vi "Start Sync.vi"(8 "error in (no error)":errorcluster, 11 "gRPC Server in":refnum<class "Query Server.lvclass">) -> (0 "error out":errorcluster, 3 "gRPC Server out":refnum<class "Query Server.lvclass">)   [LabVIEW 2019, in "Query Server.lvlib" / "Query Server.lvclass"]
uses:
  Query Server.lvclass
  gRPC lvSupport/Server API/typeDefs/grpcId.ctl
  Query Server.lvclass/Query Server.ctl
  RPC Messages/ServerEvent/ServerEvent_Data.ctl
  gRPC lvSupport/gprc-lvsupport.lvlib
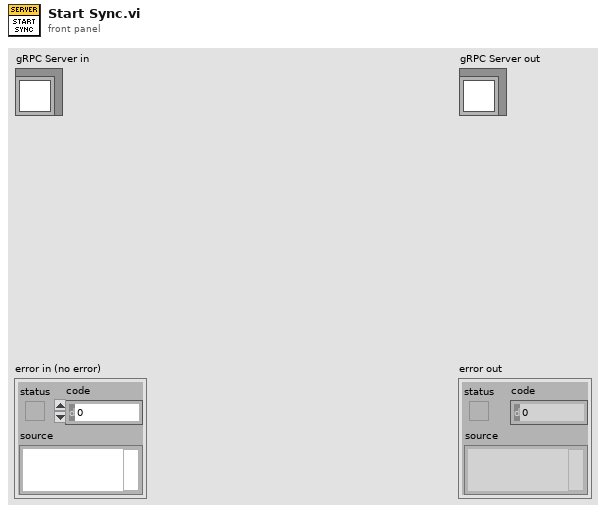
[diagram p1: front panel]
types:
  T1 = typedef "Query Server.lvlib/gprc-lvsupport.lvlib/grpcId.ctl" = u64
  T2 = typedef "Query Server.lvlib/Query Server.lvclass/ServerEvent_Data.ctl" = cluster{"eventData":string, "serverId":i32, "status":i32}
  T3 = typedef "Query Server.lvlib/Query Server.lvclass/Server gRPC UEs.ctl" = cluster{"Generic Method Event":refnum<user-event>}
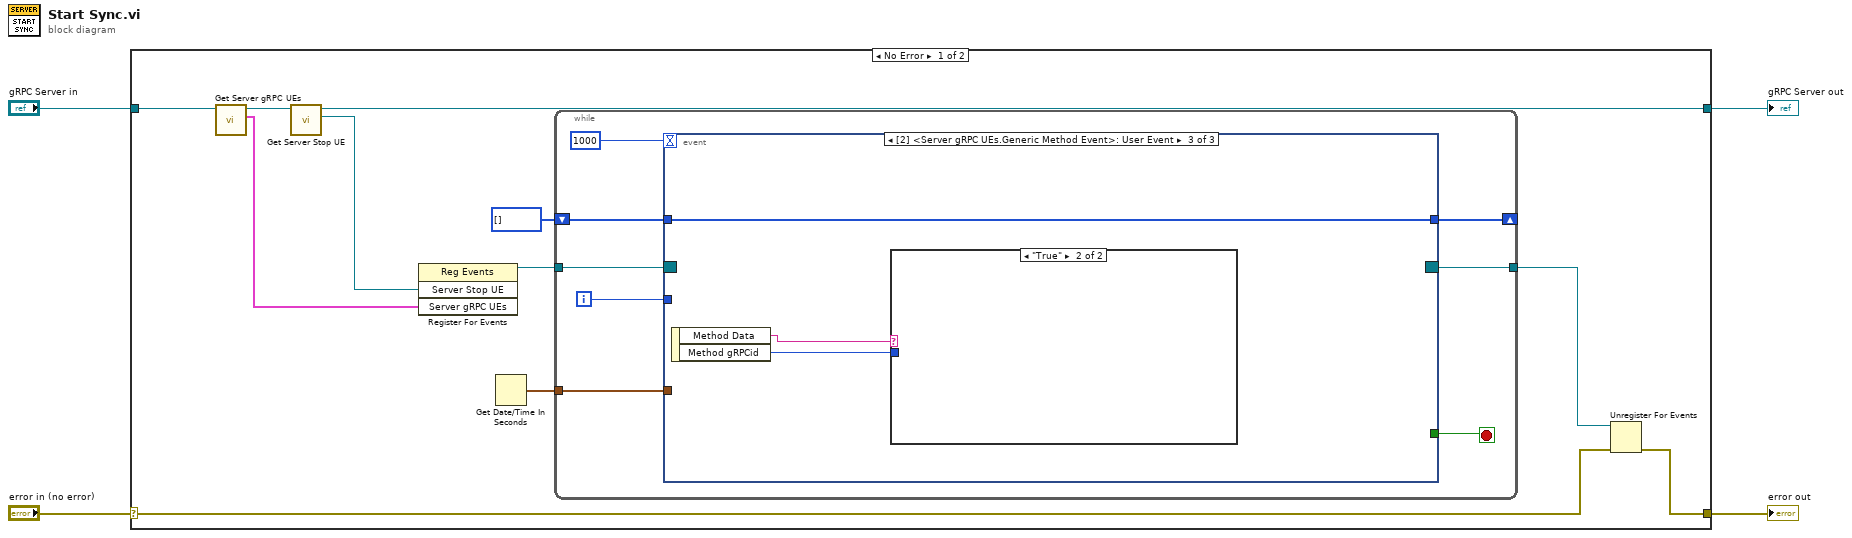
[diagram p0: block diagram]
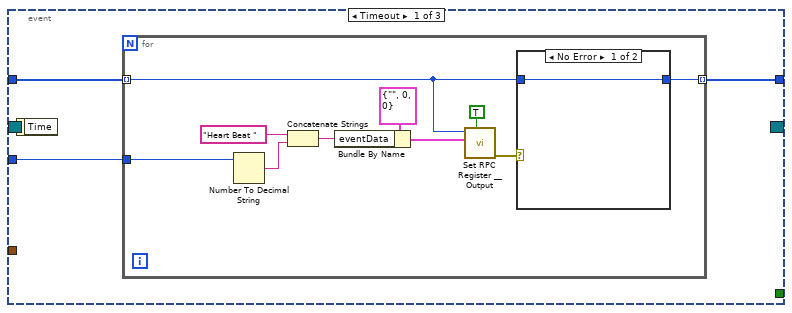
[diagram p2: hidden frame]
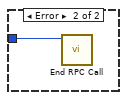
[diagram p3: hidden frame]
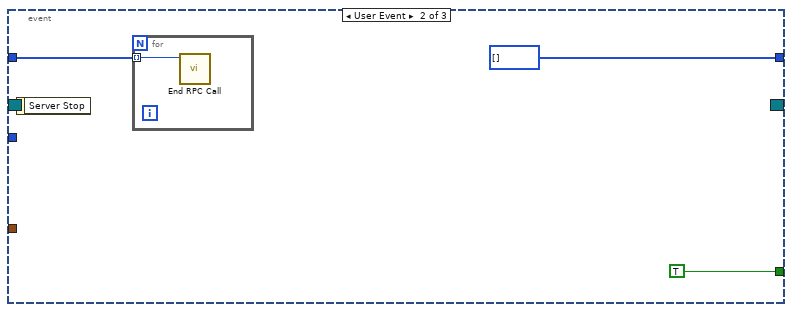
[diagram p4: hidden frame]
diagram:
  n1 = case shown="No Error" "error in (no error)" {
    selector: "error in (no error)" -> [w8 w47]
    tunnel: [w7 w47] -> w3
    tunnel: [w11 w46] -> w1
    tunnel: "gRPC Server in" -> [w15 w46]
    frame No Error {
      n2 = call "Get Server gRPC UEs.vi"("OOP Server in"=w15) -> ("Server gRPC UEs"=w12:T3, "OOP Server out"=w14:refnum<class "Query Server.lvclass">)  [unwired: 9 in]
      n3 = call "Get Server Stop UE.vi"("OOP Server in"=w14) -> ("Server Stop UE"=w13:refnum<user-event>, "OOP Server out"=w11:refnum<class "Query Server.lvclass">)  [unwired: 9 in]
      n4 = register-events(w13, w12) -> (reference out=w10:refnum<event-registration>)  [unwired: 2 in, 1 out]
      n5 = Get Date/Time In Seconds() -> (seconds since 1Jan1904=w6:timestamp)
      n6 = while {
        tunnel: w10 -> [w23]
        tunnel: [w21] -> w9
        shift-right: [w19] -> _
        shift-left: T1[] [] -> [w18]
        tunnel: w6 -> [w16]
        i -> [w17]
        stop <- w22 stop-if-true
        n7 = event "RPC Methods Event Structure" shown="[2] <Server gRPC UEs.Generic Method Event>: User Event" {
          selector: w23 -> [_ _ _]
          dyn-events: [_ _ _] -> w21
          timeout: 1000 -> [_ _ _]
          tunnel: [_ TRUE _] -> w22
          tunnel: [w24 T1[] [] w45] -> w19
          tunnel: w18 -> [w26 w40 w45]
          tunnel: w17 -> [w25 _ _]
          tunnel: w16 -> [_ _ _]
          event Timeout {
            n8 = event-data() -> ()  [unwired: 1 in, 1 out]
            n9 = for {
              tunnel: w26 -> [w30] mode=indexing
              tunnel: w25 -> [w31]
              tunnel: [w28] -> w24 mode=indexing
              n10 = Number To Decimal String(number=w31) -> (decimal integer string=w36:string)  [unwired: 1 in]
              n11 = Concatenate Strings("Heart Beat " ("eventdata"), w36) -> (w34:string)
              n12 = Bundle By Name(cluster=T2 {"eventData"="", "serverId"=0, "status"=0} ("Message Data"), "eventData"=w34) -> (w32:T2)
              n13 = call "Set RPC Register __Output.vi"("Streeming? (F)"=TRUE, "Message Data"=w32, "gRPCid in"=w30) -> ("error out"=w29:errorcluster)  [unwired: 8 in]
              n14 = case shown="No Error" w29 {
                tunnel: w30 -> [w37 w38]
                tunnel: [w37 _] -> w28
                frame No Error {
                }
                frame Error {
                  n15 = call "End RPC Call.vi"("gRPCid"=w38) -> ()  [unwired: 10 in, 1 out]
                }
              }
            }
          }
          event User Event {
            n16 = event-data() -> ()  [unwired: 1 in, 1 out]
            n17 = for {
              tunnel: w40 -> [w42] mode=indexing
              n18 = call "End RPC Call.vi"("gRPCid"=w42) -> ()  [unwired: 10 in, 1 out]
            }
          }
          event User Event {
            n19 = event-data() -> ("Method Data"=w44:string, "Method gRPCid"=w43:T1)  [unwired: 1 in]
            n20 = case shown="\"True\"" w44 {
              tunnel: w43 -> [_ _]
              frame "False", Default {
              }
              frame "True" {
              }
            }
          }
        }
      }
      n21 = Unregister For Events(event registration refnum=w9, error in=w8) -> (error out=w7:errorcluster)
    }
    frame Error {
    }
  }
  "error out" <- w3
  "gRPC Server out" <- w1
